vi "Seconds cals.vi"() -> ()   [LabVIEW 2014]
panel:
  out "seconds":dbl
  out "minutes":dbl
  out "hours":dbl
  in  "Numeric":dbl
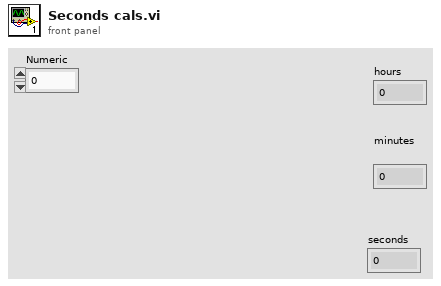
[diagram p1: front panel]
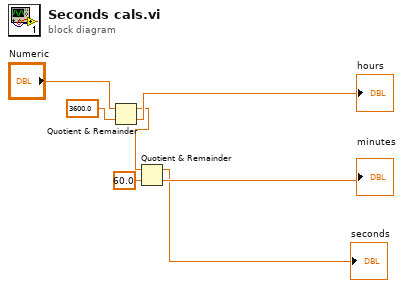
[diagram p0: block diagram]
diagram:
  n1 = Quotient & Remainder(x="Numeric", y=3600.0 ("x")) -> (x-y*floor(x/y)=w4:dbl, floor(x/y)=→"hours":dbl)
  n2 = Quotient & Remainder(x=w4, y=60.0 ("floor(x/y)")) -> (x-y*floor(x/y)=→"seconds":dbl, floor(x/y)=→"minutes":dbl)
